vi "Test Devises Status.vi"() -> (3 "subarray":string[](array[string]))   [LabVIEW 2019]
uses:
  <resource>/objmgr/nicontrollersysapi.rc
  <vilib>/nisyscfg/nisyscfg.lvlib
  <resource>/objmgr/niflexrioatomicsae.rc
  <vilib>/nisyscfg/Filter Mode.ctl
  <vilib>/nisyscfg/Close (Hardware).vi
  <vilib>/nisyscfg/Close (System).vi
  <vilib>/nisyscfg/Close (Filter).vi
panel:
  in  "error in (no error)":errorcluster
  out "error out":errorcluster
  in  "User Name":string
  in  "Password":string
  in  "Show All Network Devices":bool
  out "Resources":string[][](table)
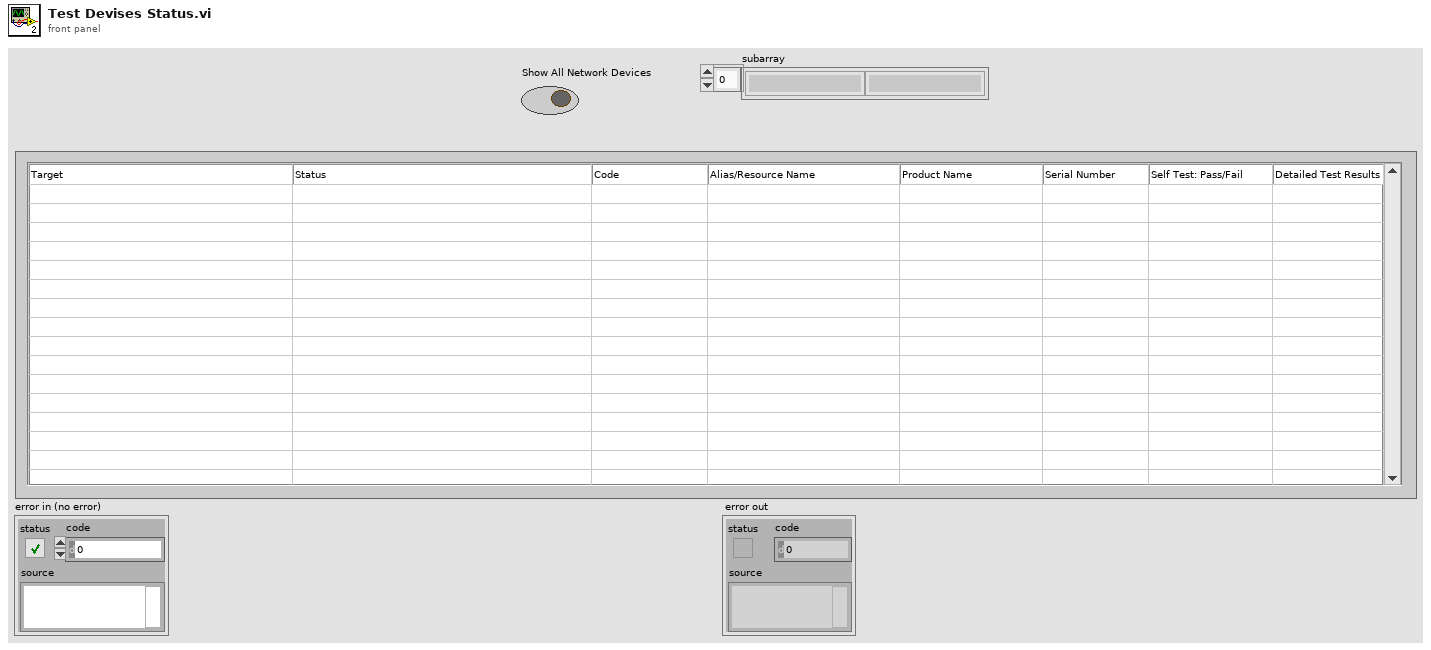
[diagram p1: front panel]
types:
  T1 = typedef "nisyscfg.lvlib/Filter Mode.ctl" = i32
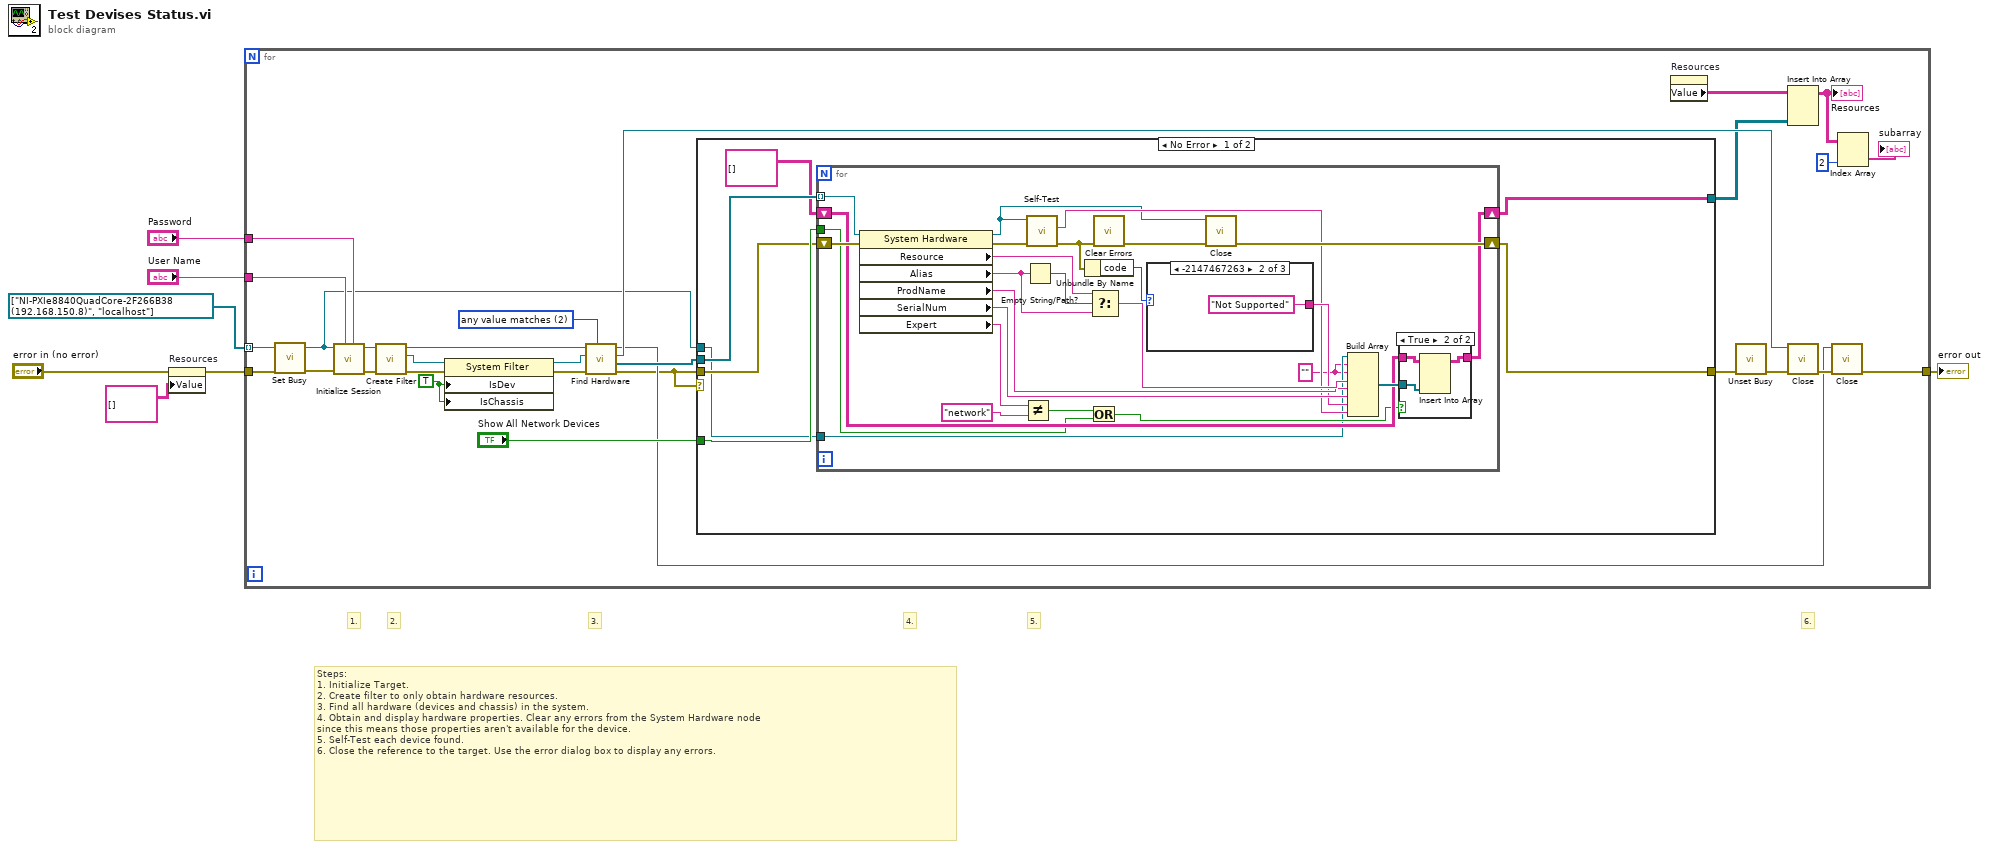
[diagram p0: block diagram]
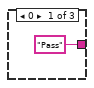
[diagram p2: hidden frame]
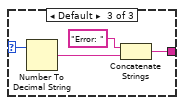
[diagram p3: hidden frame]
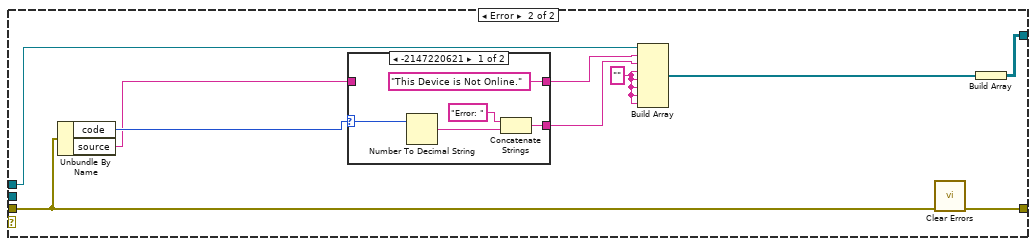
[diagram p5: hidden frame]
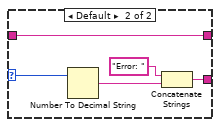
[diagram p6: hidden frame]
diagram:
  # "5."
  # "6."
  # "4."
  # "3."
  # "2."
  # "1."
  # "Steps:\n1. Initialize Target.\n2. Create filter to only obtain hardware resources.\n3. Find all hardware (devices and chassis) in the system.\n4. Obtain and display hardware properties. Clear any errors from the System Hardware node\nsince this means those properties aren't available for the device.\n5. Self-Test each device found. \n6. Close the reference to the target. Use the error dialog box to display any errors."
  n1 = property on="Resources" class="Tbl (strict)"(error in="error in (no error)", "Value"=string[][] [] ("Results")) -> (error out=w3:errorcluster)  [unwired: 1 in, 1 out]
  n2 = for {
    tunnel: "User Name" -> [w24]
    tunnel: "Password" -> [w23]
    tunnel: refnum<k21>[] ["NI-PXIe8840QuadCore-2F266B38 (192.168.150.8)", "localhost"] ("Target (localhost)") -> [w16] mode=indexing
    tunnel: w3 -> [w14]
    tunnel: [w15] -> w1
    w27 = T1 2 items=["all values match"=1, "any value matches"=2, "values do not match"=3, "all properties exist"=4] ("filter mode (all values match)")
    w22 = TRUE ("Is Chassis")
    n3 = call <vilib>:"Set Busy.vi"("error in (no error)"=w14) -> ("error out"=w13:errorcluster)  [unwired: 9 in, 1 out]
    n4 = call <vilib>:"Initialize Session.vi"("Password"=w23, "User Name"=w24, "error in (no error)"=w13, "Target (localhost)"=w16) -> ("error out"=w19:errorcluster, "Session out"=w31:refnum<k21>)  [unwired: 6 in]
    n5 = call <vilib>:"Create Filter.vi"("error in (no error)"=w19, "Session in"=w31) -> ("error out"=w33:errorcluster, "Filter out"=w32:refnum<k20>, "Session out"=w30:refnum<k21>)  [unwired: 7 in]
    n6 = property class="System Filter"(reference=w32, error in=w33, "IsDev"=w22, "IsChassis"=w22) -> (reference out=w28:refnum<k20>, error out=w29:errorcluster)
    n7 = call <vilib>:"Find Hardware.vi"("Filter Mode (all values match)"=w27, "error in (no error)"=w29, "Filter in"=w28, "Session in"=w30) -> ("error out"=w20:errorcluster, "Resources out"=w35:refnum<k20>[], "Filter out"=w25:refnum<k20>, "Session out"=w21:refnum<k21>)  [unwired: 4 out]
    n8 = case shown="No Error" w20 {
      tunnel: w35 -> [w42 _]
      tunnel: [w41 w84] -> w18
      tunnel: "Show All Network Devices" -> [w40 _]
      tunnel: [w39 w87] -> w12
      tunnel: w20 -> [w38 w79]
      tunnel: w16 -> [w37 w88]
      frame No Error {
        n9 = for {
          tunnel: w42 -> [w66] mode=indexing
          shift-right: [w68] -> w39
          shift-left: w38 -> [w60]
          shift-right: [w59] -> w41
          shift-left: string[][] [] ("Results") -> [w57]
          tunnel: w40 -> [w52]
          tunnel: w37 -> [w44]
          w43 = "" ("y")
          n10 = property class="System Hardware"(reference=w66, error in=w60) -> (reference out=w45:refnum<k20>, error out=w50:errorcluster, "Resource"=w64:string, "Alias"=w65:string, "ProdName"=w62:string, "SerialNum"=w61:string, "Expert"=w56:string)
          n11 = Not Equal?(x=w56, y="network") -> (x != y?=w53:bool)
          n12 = Empty String/Path?(string/path=w65) -> (empty?=w67:bool)
          n13 = call <vilib>:"Self-Test.vi"("error in (no error)"=w50, "Resource in"=w45) -> ("error out"=w46:errorcluster, "Detailed Result"=w47:string)  [unwired: 7 in, 1 out]
          n14 = Unbundle By Name(w46) -> ("code"=w49:i32)
          n15 = Or(x=w53, y=w52) -> (x .or. y?=w54:bool)
          n16 = Select(t=w64, s=w67, f=w65) -> (s? t:f=w63:string)
          n17 = call <vilib>:"Clear Errors.vi"("error in (no error)"=w46) -> ("error out"=w51:errorcluster)  [unwired: 5 in, 1 out]
          n18 = case shown="-2147467263" w49 {
            selector: w49 -> [_ _ w72]
            tunnel: ["Pass" ("L10n_Pass") "Not Supported" ("L10n_NotSupported") w71] -> w48
            frame 0 {
            }
            frame -2147467263 {
            }
            frame Default {
              n19 = Number To Decimal String(number=w72) -> (decimal integer string=w74:string)  [unwired: 1 in]
              n20 = Concatenate Strings("Error: " ("L10n_Error"), w74) -> (w71:string)
            }
          }
          n21 = call-poly <vilib>:"Close.vi"("error in (no error)"=w51, "Resource in"=w45) -> ("error out"=w68:errorcluster)  [unwired: 9 in]
          n22 = Build Array(w44, w43, w43, w63, w62, w61, w48, w47) -> (w58:refnum<k21>[])
          n23 = case shown="True" w54 {
            tunnel: [w75 w77] -> w59
            tunnel: w58 -> [_ w76]
            tunnel: w57 -> [w75 w78]
            frame False {
            }
            frame True {
              n24 = Insert Into Array(array=w78, new element=w76) -> (w77:string[][])  [unwired: 2 in]
            }
          }
        }
      }
      frame Error {
        w86 = ""
        n25 = Unbundle By Name(w79) -> ("code"=w83:i32, "source"=w82:string)
        n26 = case shown="-2147220621" w83 {
          selector: w83 -> [w89 w97]
          tunnel: ["This Device is Not Online." ("L10n_NotSupported") w94] -> w80
          tunnel: [w90 w95] -> w81
          tunnel: w82 -> [_ w94]
          frame -2147220621 {
            n27 = Number To Decimal String(number=w89) -> (decimal integer string=w92:string)  [unwired: 1 in]
            n28 = Concatenate Strings("Error: " ("L10n_Error"), w92) -> (w90:string)
          }
          frame Default {
            n29 = Number To Decimal String(number=w97) -> (decimal integer string=w98:string)  [unwired: 1 in]
            n30 = Concatenate Strings("Error: " ("L10n_Error"), w98) -> (w95:string)
          }
        }
        n31 = Build Array(w88, w80, w81, w86, w86, w86, w86, w86) -> (w85:refnum<k21>[])
        n32 = call <vilib>:"Clear Errors.vi"("error in (no error)"=w79) -> ("error out"=w87:errorcluster)  [unwired: 5 in, 1 out]
        n33 = Build Array(w85) -> (w84:refnum<k21>[][])
      }
    }
    n34 = property on="Resources" class="Tbl (strict)"() -> ("Value"=w17:string[][])  [unwired: 2 in, 2 out]
    n35 = call <vilib>:"Unset Busy.vi"("error in (no error)"=w12) -> ("error out"=w11:errorcluster)  [unwired: 10 in]
    n36 = Insert Into Array(array=w17, new element=w18) -> (w10:string[][])  [unwired: 2 in]
    "Resources" <- w10
    n37 = call-poly <vilib>:"Close.vi"("error in (no error)"=w11, "Filter in"=w25) -> ("error out"=w26:errorcluster)  [unwired: 9 in]
    n38 = call-poly <vilib>:"Close.vi"("error in (no error)"=w26, "Session in"=w21) -> ("error out"=w15:errorcluster)  [unwired: 9 in]
    n39 = Index Array(array=w10, index (col)=2 ("disabled index (col)")) -> (element=→"subarray":string[])  [unwired: 1 in]
  }
  "error out" <- w1
